vi "AuthorizationUpdated.vi"(8 "ErrorIn":errorcluster, 11 "ReferenceIn":refnum<class "VerticalButtonBar.lvclass">) -> (0 "ErrorOut":errorcluster, 3 "ReferenceIn":refnum<class "VerticalButtonBar.lvclass">)   [LabVIEW 2021, in "VerticalButtonBar.lvclass"]
uses:
  VerticalButtonBar.lvclass
  60d8297d-0967-4741-bf39-d248be5189e6.vi
  <vilib>/TriekselSoft/TracerLibrary/TracerLibrary/Tracer/protected/SendMessage.vi
  <vilib>/TriekselSoft/TracerLibrary/TracerLibrary/Tracer/protected/Timestamp.vi
  <vilib>/TriekselSoft/TracerLibrary/TracerLibrary/Tracer/Tracer_Level-Debug.vi
  <vilib>/TriekselSoft/TracerLibrary/TracerLibrary/Tracer/protected/Tracer_ClassAttributes.vi
  ButtonCollection/ButtonCollection.lvclass
  VerticalButtonBar.lvclass/VerticalButtonBar.ctl
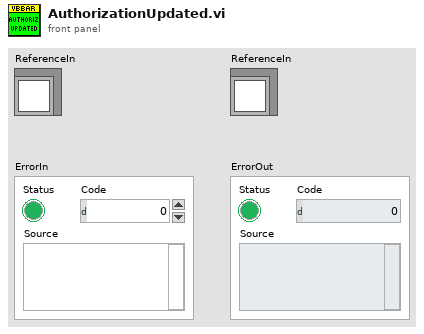
[diagram p1: front panel]
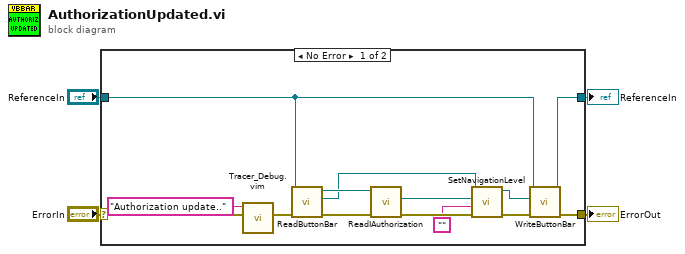
[diagram p0: block diagram]
diagram:
  n1 = case shown="No Error" "ErrorIn" {
    selector: "ErrorIn" -> [w14 w20]
    tunnel: [w15 w20] -> w3
    tunnel: [w6 w19] -> w1
    tunnel: "ReferenceIn" -> [w7 w19]
    frame No Error {
      n2 = call "Tracer_Debug.vim"("error in (no error)"=w14, "Text"="Authorization update..") -> ("error out"=w13:errorcluster)  [unwired: 9 in]
      n3 = call-dynamic "ReadButtonBar.vi"("ErrorIn"=w13, "ReferenceIn"=w7) -> ("ErrorOut"=w17:errorcluster, "ButtonBar"=w10:refnum<class "ButtonCollection.lvclass">, "ReferenceIn"=w11:refnum<class "VerticalButtonBar.lvclass">)  [unwired: 7 in]
      n4 = call-dynamic "ReadIAuthorization.vi"("ErrorIn"=w17, "ReferenceIn"=w11) -> ("ErrorOut"=w18:errorcluster, "IAuthorization"=w12:refnum<class "IAuthorization.lvclass">)  [unwired: 7 in, 1 out]
      n5 = call-dynamic "SetNavigationLevel.vi"("ErrorIn"=w18, "NavigationName"="", "Authorization"=w12, "ObjectIn"=w10) -> ("ErrorOut"=w16:errorcluster, "ObjectOut"=w8:refnum<class "ButtonCollection.lvclass">)  [unwired: 6 in]
      n6 = call-dynamic "WriteButtonBar.vi"("ErrorIn"=w16, "ButtonBar"=w8, "ReferenceIn"=w7) -> ("ErrorOut"=w15:errorcluster, "ReferenceIn"=w6:refnum<class "VerticalButtonBar.lvclass">)  [unwired: 7 in]
    }
    frame Error {
    }
  }
  "ErrorOut" <- w3
  "ReferenceIn" <- w1
